vi "Close.vi"(8 "error in (no error)":errorcluster, 11 "Total Phase Aardvark in":refnum<class "Total Phase Aardvark.lvclass">) -> (0 "error out":errorcluster, 3 "Total Phase Aardvark out":refnum<class "Total Phase Aardvark.lvclass">)   [LabVIEW 2016, in "Host Adapter.lvlib" / "Total Phase Aardvark.lvlib" / "Total Phase Aardvark.lvclass"]
uses:
  Total Phase Aardvark.lvclass
  Generic Host Adapter/Host Adapter.lvclass
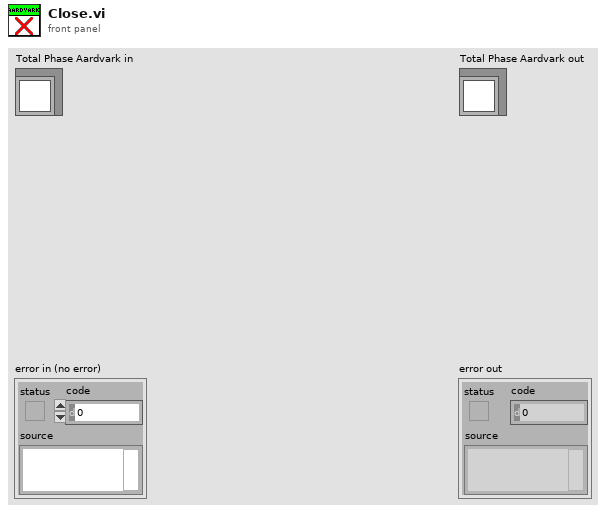
[diagram p1: front panel]
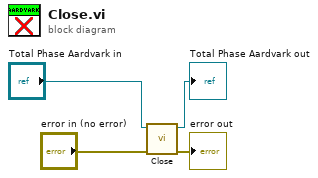
[diagram p0: block diagram]
diagram:
  n1 = call-parent "Close.vi"("error in (no error)"="error in (no error)", "Host Adapter in"="Total Phase Aardvark in") -> ("error out"=→"error out":errorcluster, "Host Adapter out"=→"Total Phase Aardvark out":refnum<class "Total Phase Aardvark.lvclass">)  [unwired: 8 in]
